vi "sub_SDR_mimo_Synchronizer.vi"(7 "decimating factor":i32=8, 10 "Received frame In":cdb[][](array[numeric])=array1x226352[226352 elements], 11 "RX Sync. Seq. (filter)":cdb[](array[numeric])) -> (0 "NextOffset":i32, 2 "Received data out":cdb[][](array[numeric]), 3 "Peak Position":i32=513)   [LabVIEW 2012]
uses:
  <vilib>/Analysis/5stat.llb/RMS (CDB).vi
  <vilib>/Analysis/2dsp.llb/1D Convolution (CDB).vi
  <vilib>/Analysis/2dsp.llb/Decimate (single shot, CDB).vi
  <vilib>/Analysis/NI_AALPro.lvlib
panel:
  out "Synchronization":dbl[](graph)
  in  "threshold":dbl=20.0
  out "Detected?":bool=TRUE
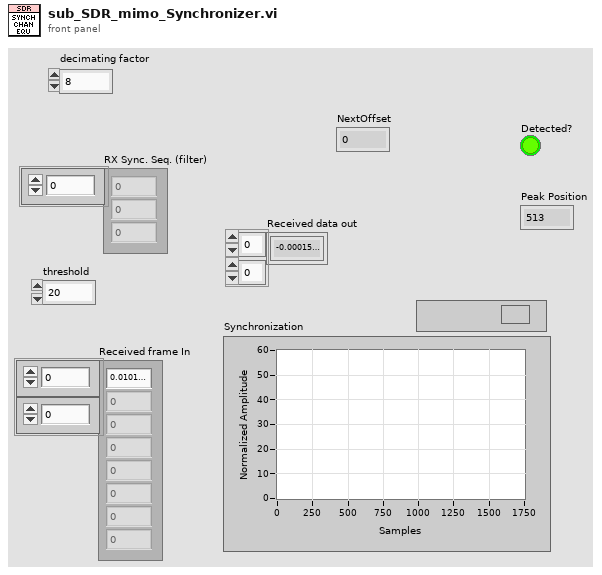
[diagram p1: front panel]
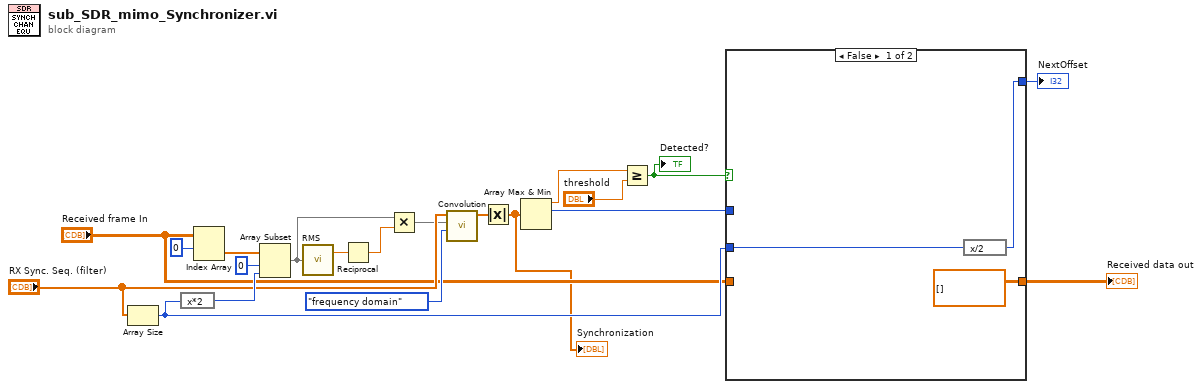
[diagram p0: block diagram]
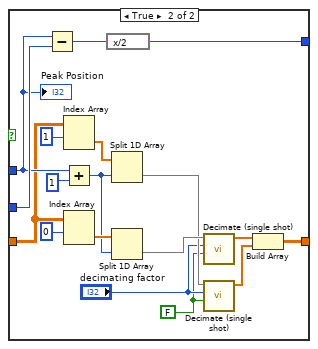
[diagram p2: hidden frame]
diagram:
  n1 = Array Size(array="RX Sync. Seq. (filter)") -> (size(s)=w9:i32)
  n2 = expression code="x*2"(w9) -> (w14:i32)
  n3 = Index Array(array="Received frame In", index (row)=0) -> (element=w5:cdb[])  [unwired: 1 in]
  n4 = Array Subset(array=w5, index=0, length=w14) -> (w7:cdb[])
  n5 = call-poly <vilib>:"RMS.vi"("X"=w7) -> ("rms value"=w13:dbl)  [unwired: 1 out]
  n6 = Reciprocal(x=w13) -> (1/x=w2:dbl)
  n7 = Multiply(x=w7, y=w2) -> (x*y=w8:cdb[])
  n8 = call-poly <vilib>:"Convolution.vi"("algorithm"=enum32{"direct", "frequency domain"}."frequency domain", "Y"=w8, "X"="RX Sync. Seq. (filter)") -> ("X * Y"=w3:cdb[])  [unwired: 7 in, 1 out]
  n9 = Absolute Value(x=w3) -> (abs(x)=w1:dbl[])
  "Synchronization" <- w1
  n10 = Array Max & Min(array=w1) -> (max value=w19:dbl, max index (indices)=w15:i32)  [unwired: 2 out]
  n11 = Greater Or Equal?(x=w19, y="threshold") -> (x >= y?=w17:bool)
  "Detected?" <- w17
  n12 = case shown="False" w17 {
    tunnel: w15 -> [_ w40]
    tunnel: w9 -> [w21 w41]
    tunnel: "Received frame In" -> [_ w34]
    tunnel: [cdb[][] [] w30] -> w16
    tunnel: [w22 w39] -> w10
    frame False {
      n13 = expression code="x/2"(w21) -> (w22:i32)
    }
    frame True {
      w25 = FALSE ("averaging")
      n14 = Subtract(x=w40, y=w41) -> (x-y=w38:i32)
      n15 = Index Array(array=w34, index (row)=1) -> (element=w32:cdb[])  [unwired: 1 in]
      n16 = Add(x=w40, y=1) -> (x+y=w31:i32)
      n17 = Index Array(array=w34, index (row)=0) -> (element=w33:cdb[])  [unwired: 1 in]
      n18 = expression code="x/2"(w38) -> (w39:i32)
      n19 = Split 1D Array(array=w32, index=w31) -> (second subarray=w27:cdb[])  [unwired: 1 out]
      n20 = Split 1D Array(array=w33, index=w31) -> (second subarray=w29:cdb[])  [unwired: 1 out]
      n21 = call-poly <vilib>:"Decimate (single shot).vi"("averaging"=w25, "decimating factor"="decimating factor", "X"=w29) -> ("Decimated Array"=w28:cdb[])  [unwired: 7 in, 1 out]
      n22 = call-poly <vilib>:"Decimate (single shot).vi"("averaging"=w25, "decimating factor"="decimating factor", "X"=w27) -> ("Decimated Array"=w24:cdb[])  [unwired: 7 in, 1 out]
      n23 = Build Array(w28, w24) -> (w30:cdb[][])
      "Peak Position" <- w40
    }
  }
  "Received data out" <- w16
  "NextOffset" <- w10
